vi "Write ADCSettings.vi"(10 "ADC Settings":T1 {"PGA Gain Coefficient" max=7}, 11 "ILC in":refnum<class "ILC.lvclass">) -> (3 "ILC out":refnum<class "ILC.lvclass">)   [LabVIEW 2015, in "ILCCommon.lvlib" / "ILC.lvclass"]
uses:
  <userlib>/Common/ILC/ILC/ILC.lvclass
  <userlib>/Common/ILC/Typedefs/ADC Settings.ctl
  <userlib>/Common/ILC/Configuration/Input Channels.ctl
  <userlib>/Common/ILC/Configuration/Scan Rates.ctl
  <userlib>/Common/ILC/ILC/ILC.lvclass/ILC.ctl
  <userlib>/Common/ILC/Configuration/ILCConfiguration.lvlib
  <userlib>/Common/ILC/Typedefs/ILCTypedefs.lvlib
panel:
  # "Gain is 2^gain_coefficient"
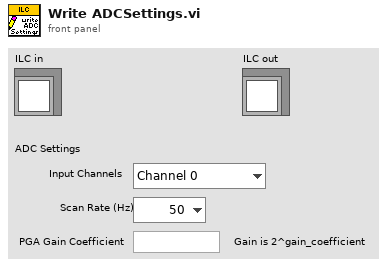
[diagram p1: front panel]
types:
  T1 = typedef "ILCCommon.lvlib/ILCTypedefs.lvlib/ADC Settings.ctl" = cluster{"Input Channels":T2, "Scan Rate (Hz) ":T3, "PGA Gain Coefficient":u8}
  T2 = typedef "ILCCommon.lvlib/ILCConfiguration.lvlib/Input Channels.ctl" = enum16{"Channel 0", "3 Channels", "5 Channels"}
  T3 = typedef "ILCCommon.lvlib/ILCConfiguration.lvlib/Scan Rates.ctl" = enum16{"50", "60", "100", "120", "200", "240", "300", "400", "480", "600", "1200", "2400", "4800"}
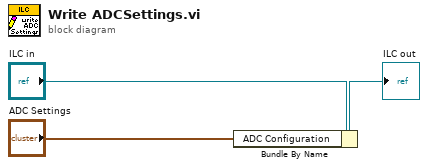
[diagram p0: block diagram]
diagram:
  n1 = Bundle By Name(cluster="ILC in", "ADC Configuration"="ADC Settings") -> (→"ILC out":refnum<class "ILC.lvclass">)
